vi "Build Constants Map.vi"(8 "error in (no error)":errorcluster, 11 "num buckets":i32=50) -> (0 "error out":errorcluster)   [LabVIEW 2013]
uses:
  Constants typedef V2.ctl
  Constants Global.vi
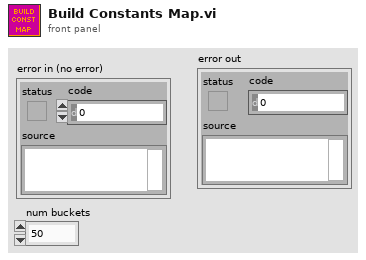
[diagram p1: front panel]
types:
  T1 = typedef "Constants typedef V2.ctl" = cluster{"Constant Name":string, "Value":dbl}
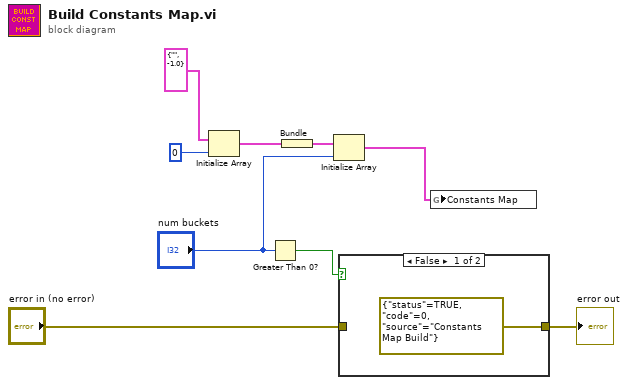
[diagram p0: block diagram]
diagram:
  n1 = Initialize Array(T1 {"Constant Name"="", "Value"=-1.0} ("Constants"), 0 ("dimension size")) -> (w4:T1[])
  n2 = Greater Than 0?(x="num buckets") -> (x > 0?=w6:bool)
  n3 = Bundle(w4) -> (w3:cluster{T1[]})  [unwired: 1 in]
  n4 = Initialize Array(w3, "num buckets") -> (w1:cluster{T1[]}[])
  n5 = case shown="False" w6 {
    tunnel: "error in (no error)" -> [_ w11]
    tunnel: [errorcluster {"status"=TRUE, "code"=0, "source"="Constants Map Build"} ("error in (no error)") w11] -> w7
    frame False {
    }
    frame True {
      # "no error"
    }
  }
  "error out" <- w7
  n6 = global write "Constants Global.vi" "Constants Map"(w1) -> ()
